vi "SRV_Build Sensor Command.vi"(0 "Sensor Config":T1={"Name"="", "A/D"=enum."Digital", "I2C Address"=0, "Register"=0, "Channel"=0, "Digital Mask"=0, "Units"="", "Sampling Mode"=enum."Polled", "Sample Period (ms)"=1000, "Formula"="", "Sensor View Config"={"Sensor Name"=enum."Gauge 01", "Minimum"=0.0, "Maximum"=10.0}, "Active"=FALSE, "PicoC Shared Var Type"=enum."Integer", "Index"=0, "Stream Multiple?"=FALSE, "Index End"=255, "Bytes"=enum."1 Byte"} {"Register" format="%.0x"; "I2C Address" format="%.0x"; "Sample Period (ms)" min=10 max=60000 step=1; "Digital Mask" format="%.0x"; "Channel" format="%.0x"}, 11 "error in (no error)":errorcluster) -> (4 "Sensor Config dup":T1={"Name"="", "A/D"=enum."Digital", "I2C Address"=0, "Register"=0, "Channel"=0, "Digital Mask"=0, "Units"="", "Sampling Mode"=enum."Polled", "Sample Period (ms)"=1000, "Formula"="", "Sensor View Config"={"Sensor Name"=enum."Gauge 01", "Minimum"=0.0, "Maximum"=10.0}, "Active"=FALSE, "PicoC Shared Var Type"=enum."Integer", "Index"=0, "Stream Multiple?"=FALSE, "Index End"=255, "Bytes"=enum."1 Byte"} {"Register" format="%.0x"; "I2C Address" format="%.0x"; "Sample Period (ms)" min=10 max=60000 step=1; "Digital Mask" format="%.0x"; "Channel" format="%.0x"}, 6 "Command":string, 8 "Active Streaming?":bool, 10 "Active Polled?":bool, 13 "Error Message":string, 14 "Constant Command":string, 15 "error out":errorcluster)   [LabVIEW 2009]
uses:
  SRV_Sensor Config Cluster.ctl
  SRV_Sensor Analog-Digital.ctl
  SRV_Sensor Sampling Mode.ctl
  SRV_Sensor View Config Cluster.ctl
  SRV_Sensors Names.ctl
  SRV_Sensor PicoC Shared Var Type.ctl
  SRV_Sensor Number of Bytes.ctl
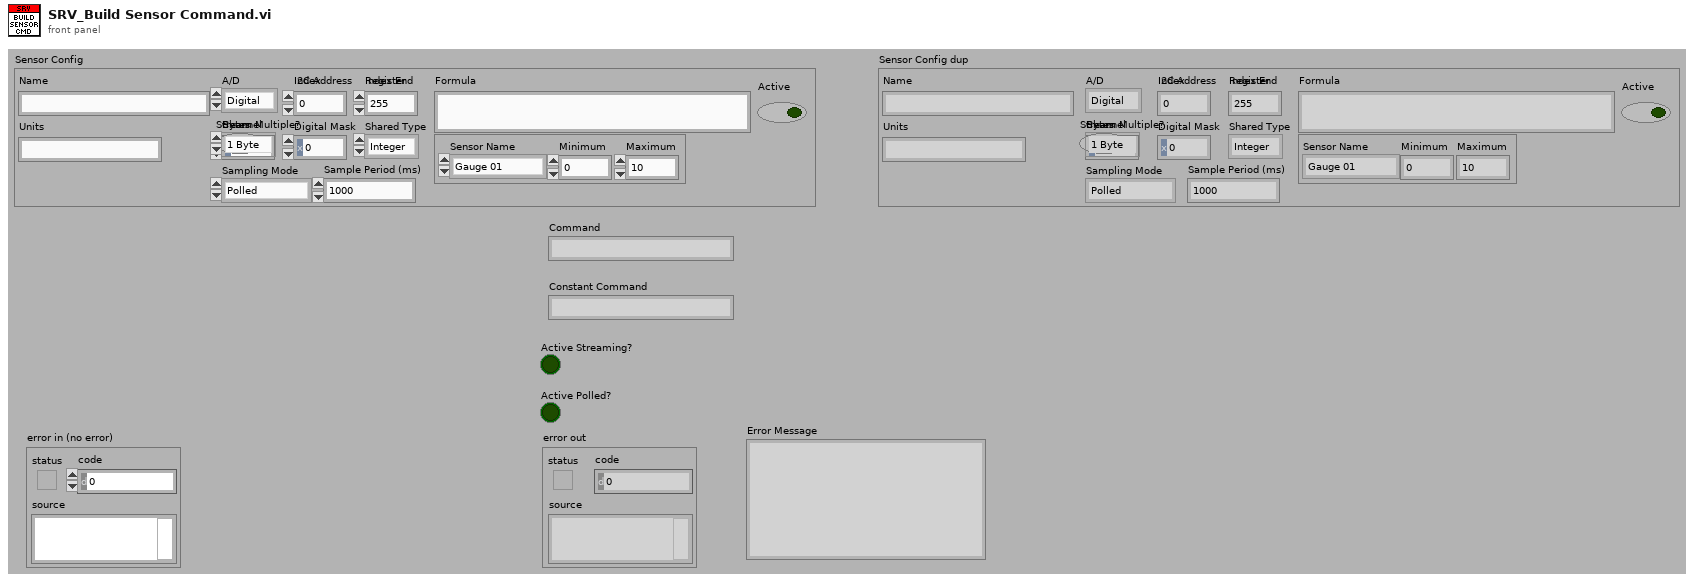
[diagram p1: front panel]
types:
  T1 = typedef "SRV_Sensor Config Cluster.ctl" = cluster{"Name":string, "A/D":T2, "I2C Address":u8, "Register":u8, "Channel":u8, "Digital Mask":u16, "Units":string, "Sampling Mode":T3, "Sample Period (ms)":u32, "Formula":string, "Sensor View Config":T4, "Active":bool, "PicoC Shared Var Type":T6, "Index":u8, "Stream Multiple?":bool, "Index End":u8, "Bytes":T7}
  T2 = typedef "SRV_Sensor Analog-Digital.ctl" = enum16{"Digital", "Analog", "PicoC Shared"}
  T3 = typedef "SRV_Sensor Sampling Mode.ctl" = enum16{"Polled", "Streaming"}
  T4 = typedef "SRV_Sensor View Config Cluster.ctl" = cluster{"Sensor Name":T5, "Minimum":dbl, "Maximum":dbl}
  T5 = typedef "SRV_Sensors Names.ctl" = enum16{"Gauge 01", "Gauge 02", "Gauge 03", "Gauge 04", "Meter 01", "Meter 02", "Meter 03", "Meter 04", "Numeric 01", "Numeric 02", "Numeric 03", "Numeric 04", "Numeric 05", "Numeric 06", "Numeric 07", "Numeric 08", "Boolean 01", "Boolean 02", "Boolean 03", "Boolean 04", "Boolean 05", "Boolean 06", "Boolean 07", "Boolean 08", "Boolean 09", "Boolean 10", "Boolean 11", "Boolean 12", "Boolean 13", "Boolean 14", "Boolean 15", "Boolean 16", "Boolean 17", "Boolean 18", "Boolean 19", "Boolean 20", "Boolean 21", "Boolean 22", "Boolean 23", "Boolean 24", "Boolean 25", "Boolean 26", "Boolean 27", "Boolean 28", "Boolean 29", "Boolean 30", "Boolean 31", "Boolean 32"}
  T6 = typedef "SRV_Sensor PicoC Shared Var Type.ctl" = enum16{"String", "Integer", "Float"}
  T7 = typedef "SRV_Sensor Number of Bytes.ctl" = enum16{"1 Byte", "2 Bytes"}
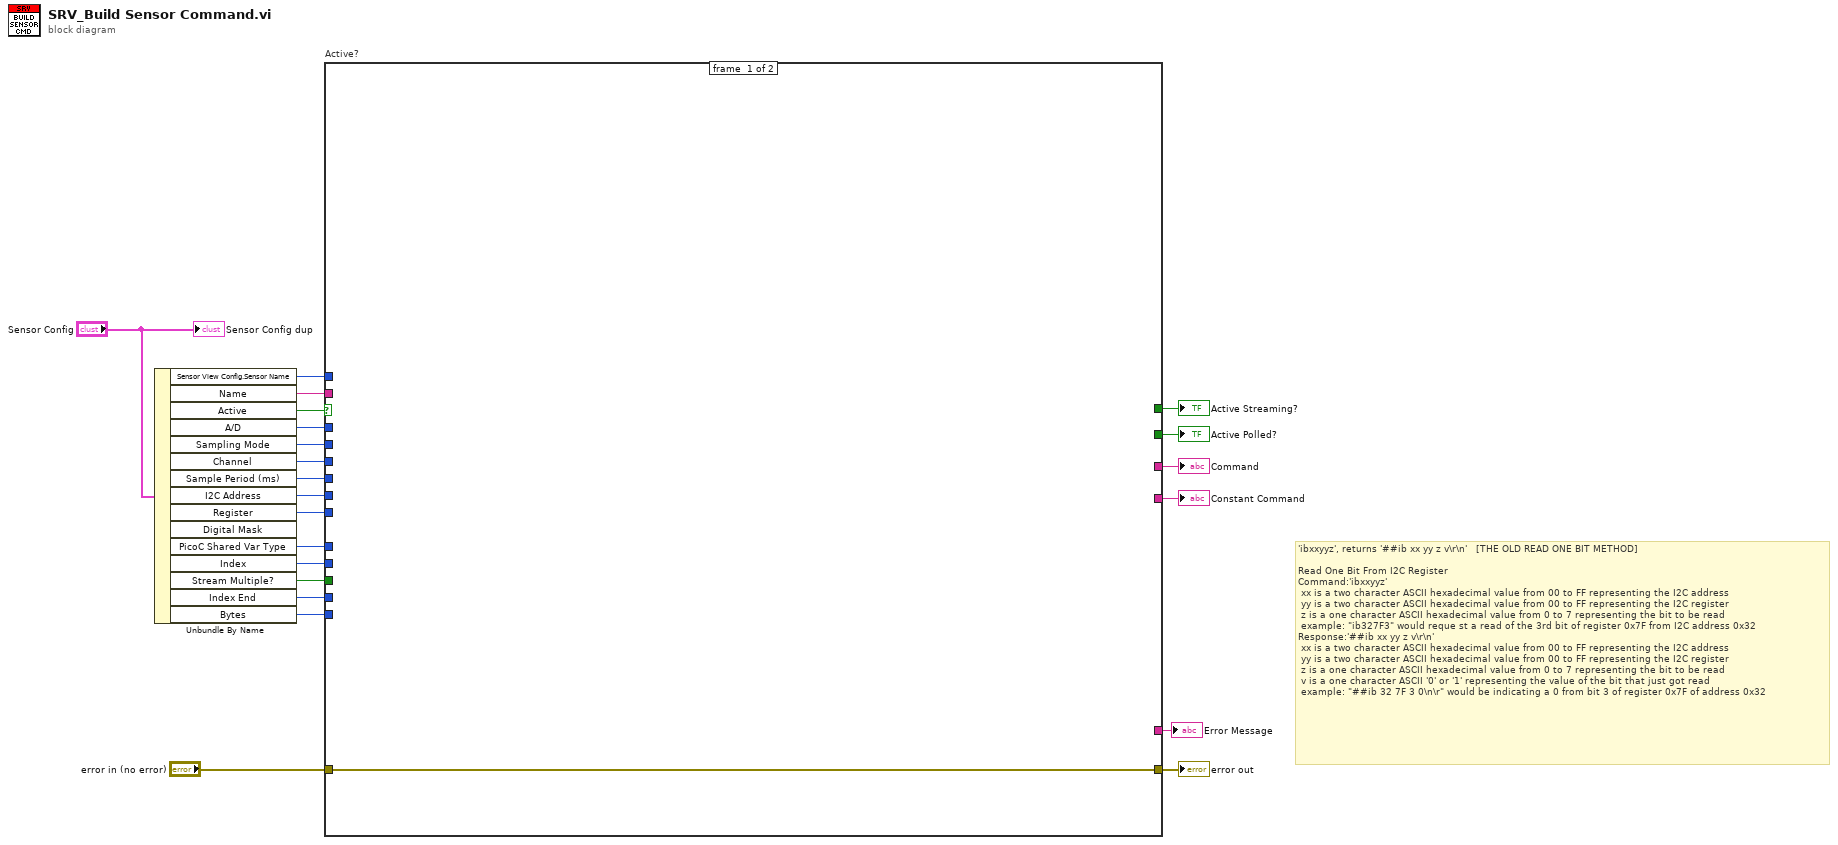
[diagram p0: block diagram]
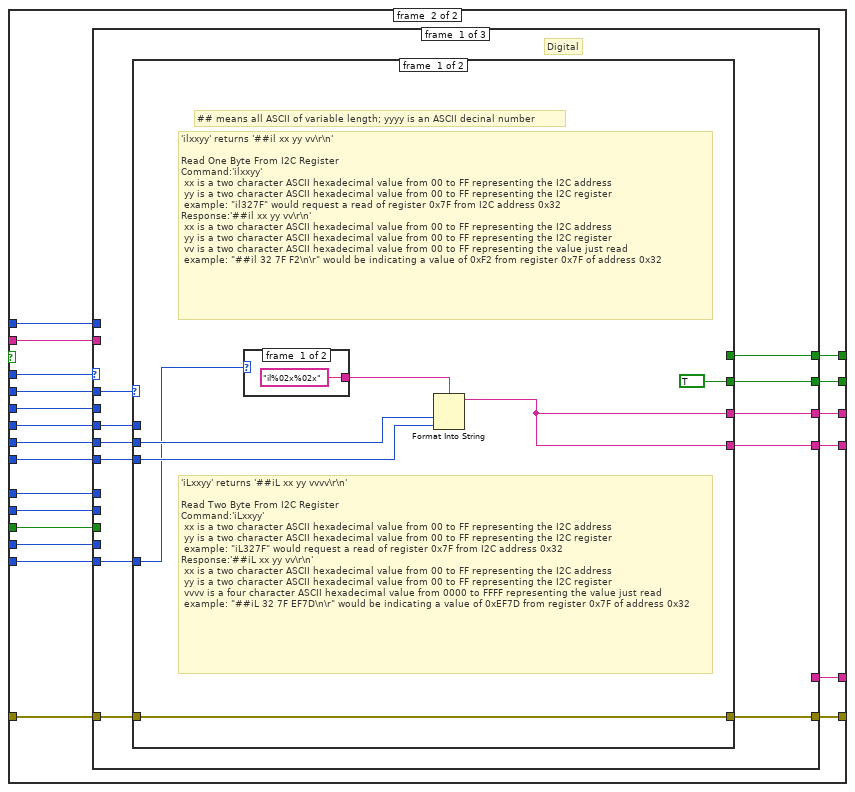
[diagram p2: hidden frame]
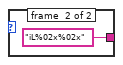
[diagram p3: hidden frame]
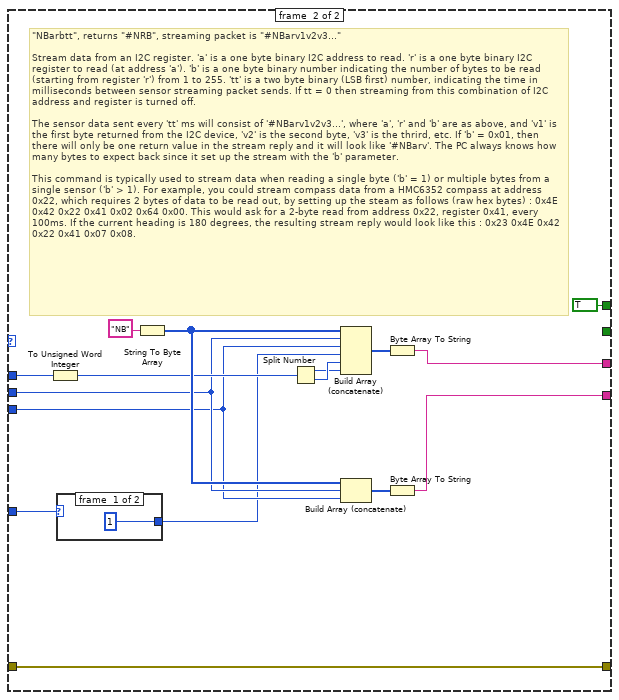
[diagram p4: hidden frame]
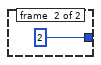
[diagram p5: hidden frame]
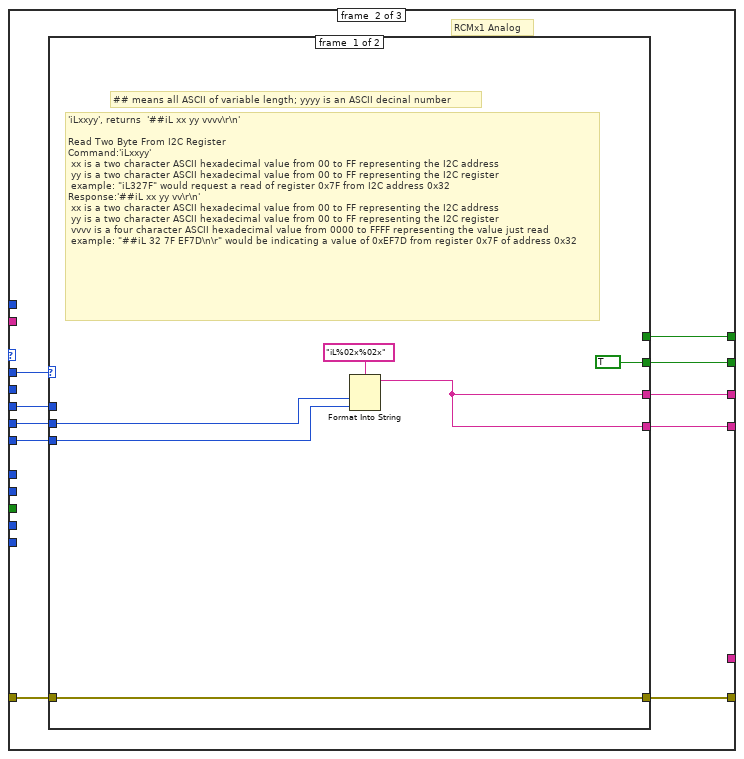
[diagram p6: hidden frame]
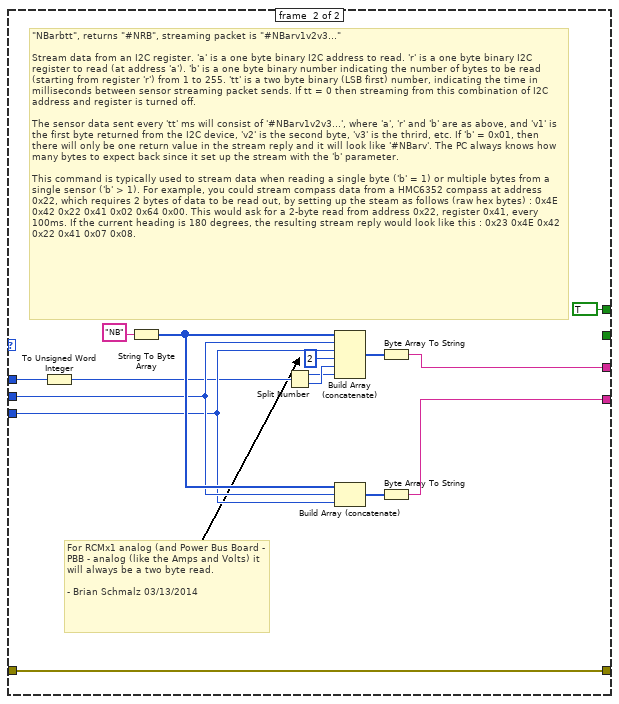
[diagram p7: hidden frame]
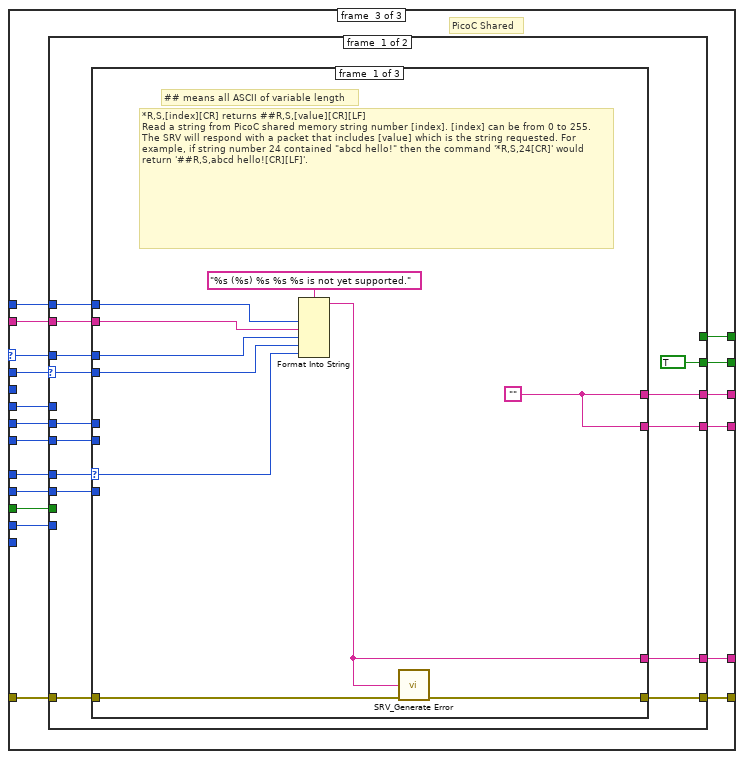
[diagram p8: hidden frame]
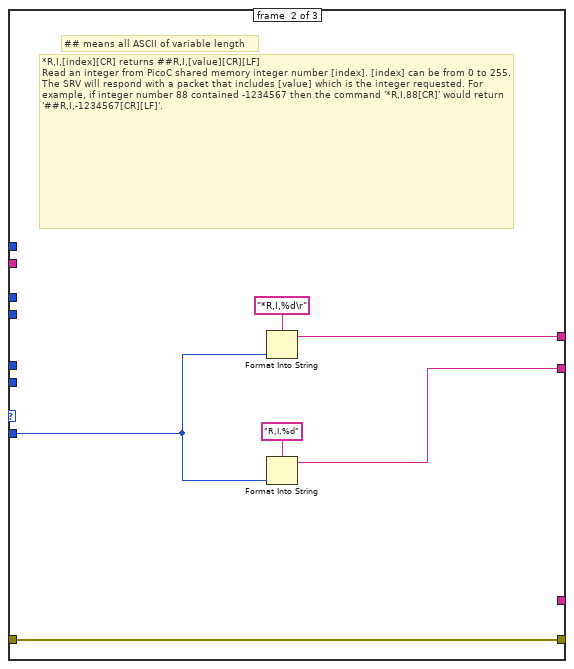
[diagram p9: hidden frame]
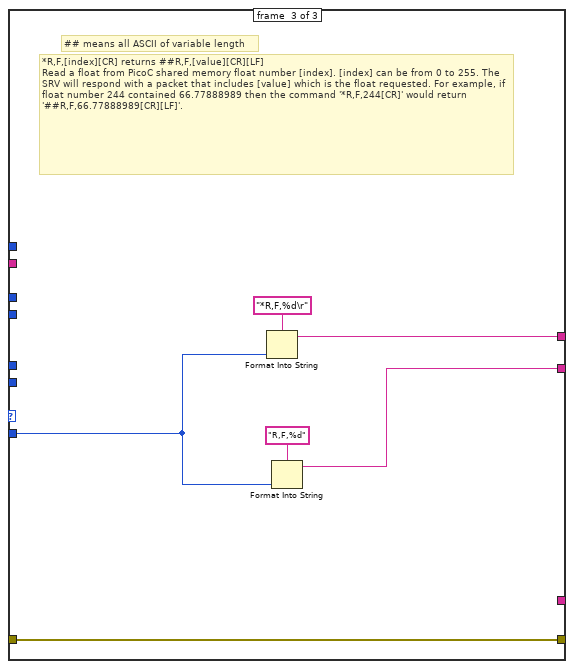
[diagram p10: hidden frame]
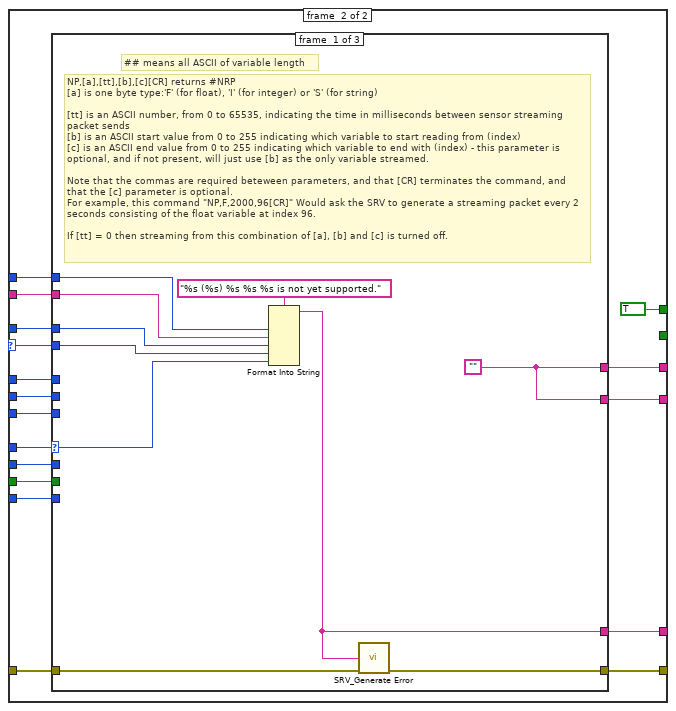
[diagram p11: hidden frame]
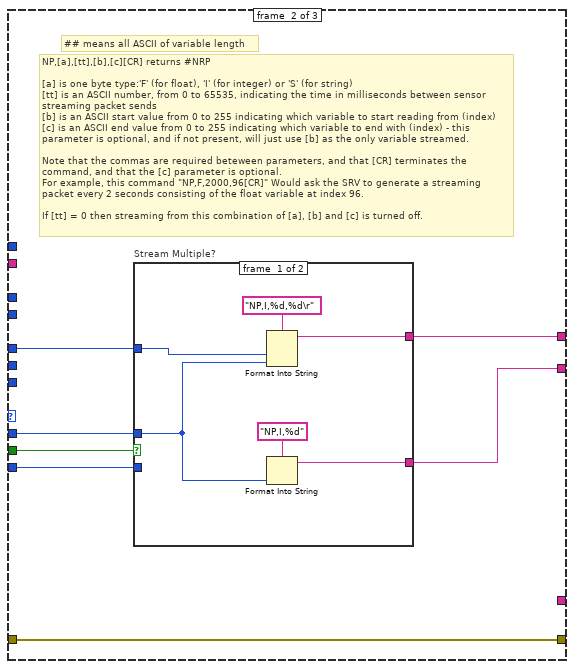
[diagram p12: hidden frame]
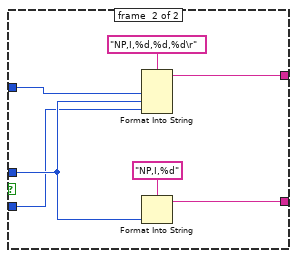
[diagram p13: hidden frame]
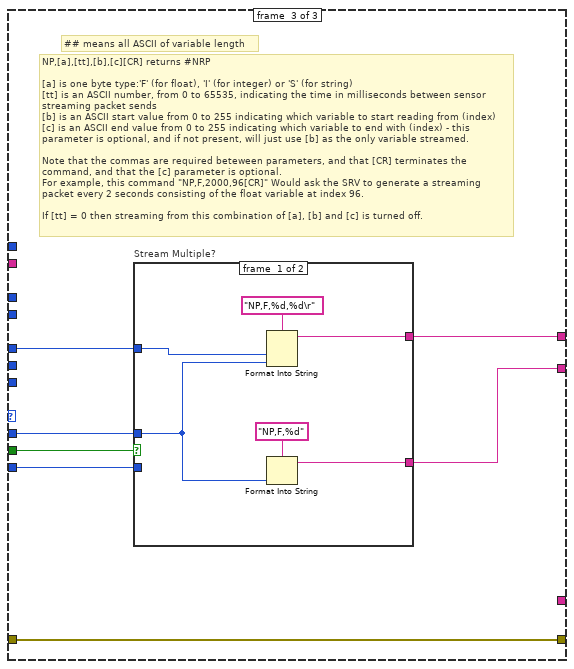
[diagram p14: hidden frame]
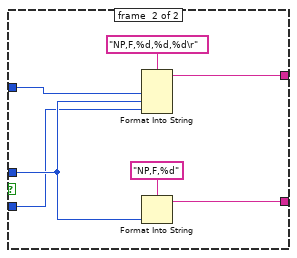
[diagram p15: hidden frame]
diagram:
  # "'ibxxyyz', returns '##ib xx yy z v\\r\\n'   [THE OLD READ ONE BIT METHOD]\n\nRead One Bit From I2C Register\nCommand:'ibxxyyz'\n xx is a two character ASCII hexadecimal value from 00 to FF representing the I2C address\n yy is a two character ASCII hexadecimal value from 00 to FF representing the I2C register\n z is a one character ASCII hexadecimal value from 0 to 7 representing the bit to be read\n example: \"ib327F3\" would reque st a read of the 3rd bit of register 0x7F from I2C address 0x32\nResponse:'##ib xx yy z v\\r\\n'\n xx is a two character ASCII hexadecimal value from 00 to FF representing the I2C address\n yy is a two character ASCII hexadecimal value from 00 to FF representing the I2C register\n z is a one character ASCII hexadecimal value from 0 to 7 representing the bit to be read\n v is a one character ASCII '0' or '1' representing the value of the bit that just got read\n example: \"##ib 32 7F 3 0\\n\\r\" would be indicating a 0 from bit 3 of register 0x7F of address 0x32"
  n1 = Unbundle By Name("Sensor Config") -> ("Sensor View Config.Sensor Name"=w2:T5, "Name"=w4:string, "Active"=w22:bool, "A/D"=w21:T2, "Sampling Mode"=w20:T3, "Channel"=w19:u8, "Sample Period (ms)"=w15:u32, "I2C Address"=w14:u8, "Register"=w13:u8, "PicoC Shared Var Type"=w8:T6, "Index"=w7:u8, "Stream Multiple?"=w6:bool, "Index End"=w5:u8, "Bytes"=w1:T7)  [unwired: 1 out]
  n2 = case "Active?" shown="True" w22 {
    tunnel: w21 -> [_ w43]
    tunnel: w20 -> [_ w42]
    tunnel: w19 -> [_ w41]
    tunnel: [_ w40] -> w17
    tunnel: w15 -> [_ w39]
    tunnel: [_ w38] -> w18
    tunnel: [_ w37] -> w16
    tunnel: w14 -> [_ w34]
    tunnel: w13 -> [_ w33]
    tunnel: "error in (no error)" -> [w23 w36]
    tunnel: [w23 w35] -> w11
    tunnel: [_ w32] -> w9
    tunnel: w8 -> [_ w31]
    tunnel: w7 -> [_ w30]
    tunnel: w6 -> [_ w29]
    tunnel: w5 -> [_ w28]
    tunnel: w4 -> [_ w27]
    tunnel: [_ w26] -> w3
    tunnel: w2 -> [_ w25]
    tunnel: w1 -> [_ w24]
    frame #0 {
    }
    frame #1 {
      n3 = case shown="\"Digital\"" w43 {
        selector: w43 -> [_ _ w120]
        tunnel: w42 -> [w54 w91 w130]
        tunnel: w41 -> [_ _ _]
        tunnel: [w48 w85 w125] -> w40
        tunnel: w39 -> [w49 w86 w126]
        tunnel: [w53 w90 w129] -> w38
        tunnel: [w52 w89 w118] -> w37
        tunnel: w36 -> [w47 w84 w124]
        tunnel: [w46 w83 w123] -> w35
        tunnel: w34 -> [w51 w88 w128]
        tunnel: w33 -> [w50 w87 w127]
        tunnel: [w45 w82 w122] -> w32
        tunnel: w31 -> [_ _ w121]
        tunnel: w30 -> [_ _ w119]
        tunnel: w29 -> [_ _ w117]
        tunnel: w28 -> [_ _ w116]
        tunnel: w27 -> [_ _ w115]
        tunnel: [_ _ w114] -> w26
        tunnel: w25 -> [_ _ w113]
        tunnel: w24 -> [w44 _ _]
        frame #0 {
          # "Digital"
          n4 = case shown="\"Streaming\"" w54 {
            tunnel: [TRUE ("Polled") _] -> w53
            tunnel: [_ TRUE ("Active Streaming?")] -> w52
            tunnel: w51 -> [w59 w67]
            tunnel: w50 -> [w58 w66]
            tunnel: w49 -> [_ w68]
            tunnel: [w57 w70] -> w48
            tunnel: w47 -> [w60 w78]
            tunnel: [w60 w78] -> w46
            tunnel: [w57 w69] -> w45
            tunnel: w44 -> [w56 w65]
            frame #0 {
              # "'iLxxyy' returns '##iL xx yy vvvv\\r\\n'\n\nRead Two Byte From I2C Register\nCommand:'iLxxyy'\n xx is a two character ASCII hexadecimal value from 00 to FF representing the I2C address\n yy is a two character ASCII hexadecimal value from 00 to FF representing the I2C register\n example: \"iL327F\" would request a read of register 0x7F from I2C address 0x32\nResponse:'##iL xx yy vv\\r\\n'\n xx is a two character ASCII hexadecimal value from 00 to FF representing the I2C address\n yy is a two character ASCII hexadecimal value from 00 to FF representing the I2C register\n vvvv is a four character ASCII hexadecimal value from 0000 to FFFF representing the value just read\n example: \"##iL 32 7F EF7D\\n\\r\" would be indicating a value of 0xEF7D from register 0x7F of address 0x32"
              # "## means all ASCII of variable length; yyyy is an ASCII decinal number"
              # "'ilxxyy' returns '##il xx yy vv\\r\\n'\n\nRead One Byte From I2C Register\nCommand:'ilxxyy'\n xx is a two character ASCII hexadecimal value from 00 to FF representing the I2C address\n yy is a two character ASCII hexadecimal value from 00 to FF representing the I2C register\n example: \"il327F\" would request a read of register 0x7F from I2C address 0x32\nResponse:'##il xx yy vv\\r\\n'\n xx is a two character ASCII hexadecimal value from 00 to FF representing the I2C address\n yy is a two character ASCII hexadecimal value from 00 to FF representing the I2C register\n vv is a two character ASCII hexadecimal value from 00 to FF representing the value just read\n example: \"##il 32 7F F2\\n\\r\" would be indicating a value of 0xF2 from register 0x7F of address 0x32"
              n5 = case shown="\"2 Bytes\"" w56 {
                tunnel: ["il%02x%02x" ("format string") "iL%02x%02x" ("format string")] -> w55
                frame #0 {
                }
                frame #1 {
                }
              }
              n6 = Format Into String(format string=w55, w59, w58) -> (resulting string=w57:string)  [unwired: 2 in, 1 out]
            }
            frame #1 {
              # "\"NBarbtt\", returns \"#NRB\", streaming packet is \"#NBarv1v2v3…\"\n\nStream data from an I2C register. 'a' is a one byte binary I2C address to read. 'r' is a one byte binary I2C register to read (at address 'a'). 'b' is a one byte binary number indicating the number of bytes to be read (starting from register 'r') from 1 to 255. 'tt' is a two byte binary (LSB first) number, indicating the time in milliseconds between sensor streaming packet sends. If tt = 0 then streaming from this combination of I2C address and register is turned off.\n\nThe sensor data sent every 'tt' ms will consist of '#NBarv1v2v3...', where 'a', 'r' and 'b' are as above, and 'v1' is the first byte returned from the I2C device, 'v2' is the second byte, 'v3' is the thrird, etc. If 'b' = 0x01, then there will only be one return value in the stream reply and it will look like '#NBarv'. The PC always knows how many bytes to expect back since it set up the stream with the 'b' parameter.\n\nThis command is typically used to stream data when reading a single byte ('b' = 1) or multiple bytes from a single sensor ('b' > 1). For example, you could stream compass data from a HMC6352 compass at address 0x22, which requires 2 bytes of data to be read out, by setting up the steam as follows (raw hex bytes) : 0x4E 0x42 0x22 0x41 0x02 0x64 0x00. This would ask for a 2-byte read from address 0x22, register 0x41, every 100ms. If the current heading is 180 degrees, the resulting stream reply would look like this : 0x23 0x4E 0x42 0x22 0x41 0x07 0x08."
              n7 = To Unsigned Word Integer(number=w68) -> (unsigned 16bit integer=w71:u16)
              n8 = case shown="\"2 Bytes\"" w65 {
                tunnel: [u8 1 ("b") u8 2 ("b")] -> w64
                frame #0 {
                }
                frame #1 {
                }
              }
              n9 = String To Byte Array(string="NB" ("format string")) -> (unsigned byte array=w72:u8[])
              n10 = Split Number(x=w71) -> (hi(x)=w74:u8, lo(x)=w75:u8)
              n11 = Build Array (concatenate)(w72, w67, w66, w64, w75, w74) -> (w76:u8[])
              n12 = Build Array (concatenate)(w72, w67, w66) -> (w73:u8[])
              n13 = Byte Array To String(unsigned byte array=w76) -> (string=w70:string)
              n14 = Byte Array To String(unsigned byte array=w73) -> (string=w69:string)
            }
          }
        }
        frame #1 {
          # "RCMx1 Analog"
          n15 = case shown="\"Streaming\"" w91 {
            tunnel: [TRUE ("Polled") _] -> w90
            tunnel: [_ TRUE ("Active Streaming?")] -> w89
            tunnel: w88 -> [w94 w102]
            tunnel: w87 -> [w93 w101]
            tunnel: w86 -> [_ w111]
            tunnel: [w92 w105] -> w85
            tunnel: w84 -> [w96 w110]
            tunnel: [w96 w110] -> w83
            tunnel: [w92 w100] -> w82
            frame #0 {
              # "## means all ASCII of variable length; yyyy is an ASCII decinal number"
              # "'iLxxyy', returns  '##iL xx yy vvvv\\r\\n'\n\nRead Two Byte From I2C Register\nCommand:'iLxxyy'\n xx is a two character ASCII hexadecimal value from 00 to FF representing the I2C address\n yy is a two character ASCII hexadecimal value from 00 to FF representing the I2C register\n example: \"iL327F\" would request a read of register 0x7F from I2C address 0x32\nResponse:'##iL xx yy vv\\r\\n'\n xx is a two character ASCII hexadecimal value from 00 to FF representing the I2C address\n yy is a two character ASCII hexadecimal value from 00 to FF representing the I2C register\n vvvv is a four character ASCII hexadecimal value from 0000 to FFFF representing the value just read\n example: \"##iL 32 7F EF7D\\n\\r\" would be indicating a value of 0xEF7D from register 0x7F of address 0x32"
              n16 = Format Into String(format string="iL%02x%02x", w94, w93) -> (resulting string=w92:string)  [unwired: 2 in, 1 out]
            }
            frame #1 {
              # "For RCMx1 analog (and Power Bus Board - PBB - analog (like the Amps and Volts) it will always be a two byte read.\n\n- Brian Schmalz 03/13/2014"
              # "\"NBarbtt\", returns \"#NRB\", streaming packet is \"#NBarv1v2v3…\"\n\nStream data from an I2C register. 'a' is a one byte binary I2C address to read. 'r' is a one byte binary I2C register to read (at address 'a'). 'b' is a one byte binary number indicating the number of bytes to be read (starting from register 'r') from 1 to 255. 'tt' is a two byte binary (LSB first) number, indicating the time in milliseconds between sensor streaming packet sends. If tt = 0 then streaming from this combination of I2C address and register is turned off.\n\nThe sensor data sent every 'tt' ms will consist of '#NBarv1v2v3...', where 'a', 'r' and 'b' are as above, and 'v1' is the first byte returned from the I2C device, 'v2' is the second byte, 'v3' is the thrird, etc. If 'b' = 0x01, then there will only be one return value in the stream reply and it will look like '#NBarv'. The PC always knows how many bytes to expect back since it set up the stream with the 'b' parameter.\n\nThis command is typically used to stream data when reading a single byte ('b' = 1) or multiple bytes from a single sensor ('b' > 1). For example, you could stream compass data from a HMC6352 compass at address 0x22, which requires 2 bytes of data to be read out, by setting up the steam as follows (raw hex bytes) : 0x4E 0x42 0x22 0x41 0x02 0x64 0x00. This would ask for a 2-byte read from address 0x22, register 0x41, every 100ms. If the current heading is 180 degrees, the resulting stream reply would look like this : 0x23 0x4E 0x42 0x22 0x41 0x07 0x08."
              n17 = To Unsigned Word Integer(number=w111) -> (unsigned 16bit integer=w99:u16)
              n18 = String To Byte Array(string="NB" ("format string")) -> (unsigned byte array=w103:u8[])
              n19 = Split Number(x=w99) -> (hi(x)=w106:u8, lo(x)=w107:u8)
              n20 = Build Array (concatenate)(w103, w102, w101, u8 2 ("b"), w107, w106) -> (w108:u8[])
              n21 = Build Array (concatenate)(w103, w102, w101) -> (w104:u8[])
              n22 = Byte Array To String(unsigned byte array=w108) -> (string=w105:string)
              n23 = Byte Array To String(unsigned byte array=w104) -> (string=w100:string)
            }
          }
        }
        frame #2 {
          # "PicoC Shared"
          n24 = case shown="\"Streaming\"" w130 {
            selector: w130 -> [w137 w177]
            tunnel: [TRUE ("Polled") _] -> w129
            tunnel: w128 -> [w143 w183]
            tunnel: w127 -> [w142 w182]
            tunnel: w126 -> [_ w172]
            tunnel: [w134 w174] -> w125
            tunnel: w124 -> [w141 w181]
            tunnel: [w140 w180] -> w123
            tunnel: [w135 w175] -> w122
            tunnel: w121 -> [w139 w179]
            tunnel: w120 -> [w138 w178]
            tunnel: w119 -> [w136 w176]
            tunnel: [_ TRUE ("Active Streaming?")] -> w118
            tunnel: w117 -> [_ w171]
            tunnel: w116 -> [_ w170]
            tunnel: w115 -> [w133 w169]
            tunnel: [w132 w168] -> w114
            tunnel: w113 -> [w131 w167]
            frame #0 {
              n25 = case shown="\"Integer\"" w139 {
                selector: w139 -> [w152 _ _]
                tunnel: w143 -> [_ _ _]
                tunnel: w142 -> [_ _ _]
                tunnel: [w149 w159 w165] -> w134
                tunnel: w141 -> [w151 w158 w164]
                tunnel: [w150 w158 w164] -> w140
                tunnel: w138 -> [w148 _ _]
                tunnel: w137 -> [w153 _ _]
                tunnel: w136 -> [_ w155 w162]
                tunnel: [w149 w156 w161] -> w135
                tunnel: w133 -> [w146 _ _]
                tunnel: [w147 _ _] -> w132
                tunnel: w131 -> [w145 _ _]
                frame #0 {
                  w149 = ""
                  # "## means all ASCII of variable length"
                  # "*R,S,[index][CR] returns ##R,S,[value][CR][LF]\nRead a string from PicoC shared memory string number [index]. [index] can be from 0 to 255. The SRV will respond with a packet that includes [value] which is the string requested. For example, if string number 24 contained \"abcd hello!\" then the command '*R,S,24[CR]' would return '##R,S,abcd hello![CR][LF]'."
                  n26 = Format Into String(format string="%s (%s) %s %s %s is not yet supported.", w145, w146, w148, w153, w152) -> (resulting string=w147:string)  [unwired: 2 in, 1 out]
                  n27 = call "SRV_Generate Error.vi"("Message"=w147, "error in (no error)"=w151) -> ("error out"=w150:errorcluster)  [unwired: 13 in]
                }
                frame #1 {
                  # "## means all ASCII of variable length"
                  # "*R,I,[index][CR] returns ##R,I,[value][CR][LF]\nRead an integer from PicoC shared memory integer number [index]. [index] can be from 0 to 255. The SRV will respond with a packet that includes [value] which is the integer requested. For example, if integer number 88 contained -1234567 then the command '*R,I,88[CR]' would return '##R,I,-1234567[CR][LF]'."
                  n28 = Format Into String(format string="*R,I,%d\r", w155) -> (resulting string=w159:string)  [unwired: 2 in, 1 out]
                  n29 = Format Into String(format string="R,I,%d", w155) -> (resulting string=w156:string)  [unwired: 2 in, 1 out]
                }
                frame #2 {
                  # "## means all ASCII of variable length"
                  # "*R,F,[index][CR] returns ##R,F,[value][CR][LF]\nRead a float from PicoC shared memory float number [index]. [index] can be from 0 to 255. The SRV will respond with a packet that includes [value] which is the float requested. For example, if float number 244 contained 66.77888989 then the command '*R,F,244[CR]' would return '##R,F,66.77888989[CR][LF]'."
                  n30 = Format Into String(format string="*R,F,%d\r", w162) -> (resulting string=w165:string)  [unwired: 2 in, 1 out]
                  n31 = Format Into String(format string="R,F,%d", w162) -> (resulting string=w161:string)  [unwired: 2 in, 1 out]
                }
              }
            }
            frame #1 {
              n32 = case shown="\"Float\"" w179 {
                selector: w179 -> [w191 _ _]
                tunnel: w183 -> [_ _ _]
                tunnel: w182 -> [_ _ _]
                tunnel: [w188 w200 w220] -> w174
                tunnel: w181 -> [w190 w199 w219]
                tunnel: [w189 w199 w219] -> w180
                tunnel: w178 -> [w187 _ _]
                tunnel: w177 -> [w192 _ _]
                tunnel: w176 -> [_ w197 w217]
                tunnel: [w188 w198 w218] -> w175
                tunnel: w172 -> [_ w196 w216]
                tunnel: w171 -> [_ w195 w215]
                tunnel: w170 -> [_ w194 w214]
                tunnel: w169 -> [w185 _ _]
                tunnel: [w186 _ _] -> w168
                tunnel: w167 -> [w184 _ _]
                frame #0 {
                  w188 = ""
                  # "## means all ASCII of variable length"
                  # "NP,[a],[tt],[b],[c][CR] returns #NRP\n[a] is one byte type:'F' (for float), 'I' (for integer) or 'S' (for string)\n\n[tt] is an ASCII number, from 0 to 65535, indicating the time in milliseconds between sensor streaming packet sends\n[b] is an ASCII start value from 0 to 255 indicating which variable to start reading from (index)\n[c] is an ASCII end value from 0 to 255 indicating which variable to end with (index) - this parameter is optional, and if not present, will just use [b] as the only variable streamed.\n\nNote that the commas are required beteween parameters, and that [CR] terminates the command, and that the [c] parameter is optional.\nFor example, this command \"NP,F,2000,96[CR]\" Would ask the SRV to generate a streaming packet every 2 seconds consisting of the float variable at index 96.\n\nIf [tt] = 0 then streaming from this combination of [a], [b] and [c] is turned off."
                  n33 = Format Into String(format string="%s (%s) %s %s %s is not yet supported.", w184, w185, w187, w192, w191) -> (resulting string=w186:string)  [unwired: 2 in, 1 out]
                  n34 = call "SRV_Generate Error.vi"("Message"=w186, "error in (no error)"=w190) -> ("error out"=w189:errorcluster)  [unwired: 13 in]
                }
                frame #1 {
                  # "## means all ASCII of variable length"
                  # "NP,[a],[tt],[b],[c][CR] returns #NRP\n\n[a] is one byte type:'F' (for float), 'I' (for integer) or 'S' (for string)\n[tt] is an ASCII number, from 0 to 65535, indicating the time in milliseconds between sensor streaming packet sends\n[b] is an ASCII start value from 0 to 255 indicating which variable to start reading from (index)\n[c] is an ASCII end value from 0 to 255 indicating which variable to end with (index) - this parameter is optional, and if not present, will just use [b] as the only variable streamed.\n\nNote that the commas are required beteween parameters, and that [CR] terminates the command, and that the [c] parameter is optional.\nFor example, this command \"NP,F,2000,96[CR]\" Would ask the SRV to generate a streaming packet every 2 seconds consisting of the float variable at index 96.\n\nIf [tt] = 0 then streaming from this combination of [a], [b] and [c] is turned off."
                  n35 = case "Stream Multiple?" shown="False" w195 {
                    tunnel: [w205 w212] -> w200
                    tunnel: [w203 w210] -> w198
                    tunnel: w197 -> [w202 w209]
                    tunnel: w196 -> [w201 w208]
                    tunnel: w194 -> [_ w207]
                    frame #0 {
                      n36 = Format Into String(format string="NP,I,%d,%d\r", w201, w202) -> (resulting string=w205:string)  [unwired: 2 in, 1 out]
                      n37 = Format Into String(format string="NP,I,%d", w202) -> (resulting string=w203:string)  [unwired: 2 in, 1 out]
                    }
                    frame #1 {
                      n38 = Format Into String(format string="NP,I,%d,%d,%d\r", w208, w209, w207) -> (resulting string=w212:string)  [unwired: 2 in, 1 out]
                      n39 = Format Into String(format string="NP,I,%d", w209) -> (resulting string=w210:string)  [unwired: 2 in, 1 out]
                    }
                  }
                }
                frame #2 {
                  # "## means all ASCII of variable length"
                  # "NP,[a],[tt],[b],[c][CR] returns #NRP\n\n[a] is one byte type:'F' (for float), 'I' (for integer) or 'S' (for string)\n[tt] is an ASCII number, from 0 to 65535, indicating the time in milliseconds between sensor streaming packet sends\n[b] is an ASCII start value from 0 to 255 indicating which variable to start reading from (index)\n[c] is an ASCII end value from 0 to 255 indicating which variable to end with (index) - this parameter is optional, and if not present, will just use [b] as the only variable streamed.\n\nNote that the commas are required beteween parameters, and that [CR] terminates the command, and that the [c] parameter is optional.\nFor example, this command \"NP,F,2000,96[CR]\" Would ask the SRV to generate a streaming packet every 2 seconds consisting of the float variable at index 96.\n\nIf [tt] = 0 then streaming from this combination of [a], [b] and [c] is turned off."
                  n40 = case "Stream Multiple?" shown="False" w215 {
                    tunnel: [w225 w232] -> w220
                    tunnel: [w223 w230] -> w218
                    tunnel: w217 -> [w222 w229]
                    tunnel: w216 -> [w221 w228]
                    tunnel: w214 -> [_ w227]
                    frame #0 {
                      n41 = Format Into String(format string="NP,F,%d,%d\r", w221, w222) -> (resulting string=w225:string)  [unwired: 2 in, 1 out]
                      n42 = Format Into String(format string="NP,F,%d", w222) -> (resulting string=w223:string)  [unwired: 2 in, 1 out]
                    }
                    frame #1 {
                      n43 = Format Into String(format string="NP,F,%d,%d,%d\r", w228, w229, w227) -> (resulting string=w232:string)  [unwired: 2 in, 1 out]
                      n44 = Format Into String(format string="NP,F,%d", w229) -> (resulting string=w230:string)  [unwired: 2 in, 1 out]
                    }
                  }
                }
              }
            }
          }
        }
      }
    }
  }
  "Active Polled?" <- w18
  "Command" <- w17
  "Active Streaming?" <- w16
  "error out" <- w11
  "Constant Command" <- w9
  "Error Message" <- w3
  "Sensor Config dup" <- "Sensor Config"
